vi "parabola -- complex.vi"(8 "n":i32, 9 "curvature":cdb, 10 "slope":cdb, 11 "intercept":cdb) -> (0 "parabola":cdb, 1 "tangent":cdb)   [LabVIEW 2020]
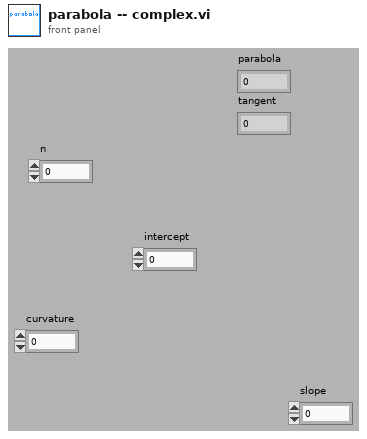
[diagram p1: front panel]
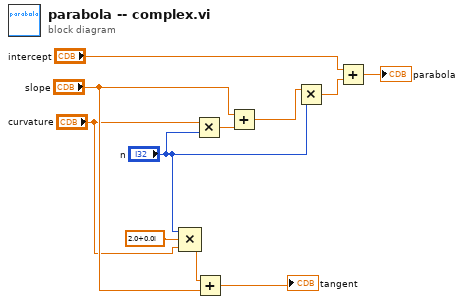
[diagram p0: block diagram]
diagram:
  n1 = Compound Arithmetic op=MULTIPLY("n", cdb 2.0+0.0i ("x"), "curvature") -> (w6:cdb)
  n2 = Multiply(x="curvature", y="n") -> (x*y=w11:cdb)
  n3 = Add(x=w6, y="slope") -> (x+y=→"tangent":cdb)
  n4 = Add(x="slope", y=w11) -> (x+y=w10:cdb)
  n5 = Multiply(x=w10, y="n") -> (x*y=w9:cdb)
  n6 = Add(x="intercept", y=w9) -> (x+y=→"parabola":cdb)
